vi "DriveStateController.vi"(1 "Selected State (In)":string) -> (0 "Selected State (Out)":string)   [LabVIEW 2019]
doc: "This VI performs all of the calculations and decisions related to the swerve drive."
uses:
  <vilib>/Rock Robotics/WPI/DriverStation/WPI_DriverStationRobotMode2.ctl
  dsinstructions.vi
  constants.vi
  dsdata.vi
  sensors.vi
  outputs.vi
panel:
  in  "Deceleration Hysteresis (ms)":u32
  in  "Driver Profiles":T1(array[cluster])=[{"Strafe Deadband"=0.08, "Rotation Deadband"=0.15, "Strafe Scaling"=3.0, "Rotation Scaling"=2.5}, {"Strafe Deadband"=0.08, "Rotation Deadband"=0.15, "Strafe Scaling"=2.0, "Rotation Scaling"=2.5}, {"Strafe Deadband"=0.08, "Rotation Deadband"=0.15, "Strafe Scaling"=2.0, "Rotation Scaling"=2.5}, {"Strafe Deadband"=0.08, "Rotation Deadband"=0.15, "Strafe Scaling"=2.0, "Rotation Scaling"=2.5}] {"Rotation Scaling" min=1.0 max=4.0 scale=1.0..4.0; "Strafe Scaling" min=1.0 max=4.0 scale=1.0..4.0; "Rotation Deadband" min=0.0 max=0.4 scale=0.0..0.4; "Strafe Deadband" min=0.0 max=0.4 scale=0.0..0.4}
  out "Heading Control":bool
  in  "Heading Lock Strafe Deadband (ft/s)":dbl=1.0
  in  "PID Tuning Heading Lock":T2={"Kp"=0.009, "Ki"=0.0, "Kd"=0.0001, "N-Diff"=5, "N-Int"=10, "Int Error Window"=30.0, "Max Ouput"=1.0, "Min Output"=-1.0} {"Int Error Window" min=0.0; "N-Int" min=2; "N-Diff" min=2; "Kd" min=0.0; "Ki" min=0.0; "Kp" min=0.0}
  in  "Manually Disable Heading Lock":bool
  in  "PID Tuning Feeder Station":T2={"Kp"=0.01, "Ki"=0.01, "Kd"=9e-05, "N-Diff"=10, "N-Int"=10, "Int Error Window"=30.0, "Max Ouput"=1.0, "Min Output"=-1.0} {"Int Error Window" min=0.0; "N-Int" min=2; "N-Diff" min=2; "Kd" min=0.0; "Ki" min=0.0; "Kp" min=0.0}
  out "Heading Controller Summary":T3(graph)
  in  "PID Tuning Auto Targeting":T2={"Kp"=0.01, "Ki"=0.01, "Kd"=9e-05, "N-Diff"=10, "N-Int"=10, "Int Error Window"=30.0, "Max Ouput"=1.0, "Min Output"=-1.0} {"Int Error Window" min=0.0; "N-Int" min=2; "N-Diff" min=2; "Kd" min=0.0; "Ki" min=0.0; "Kp" min=0.0}
  in  "Manual Fudge Factor (deg)":dbl=5.0
  in  "Plot Heading PID":bool
  in  "Sync Driver Profile":bool
  out "Selected Driver":string
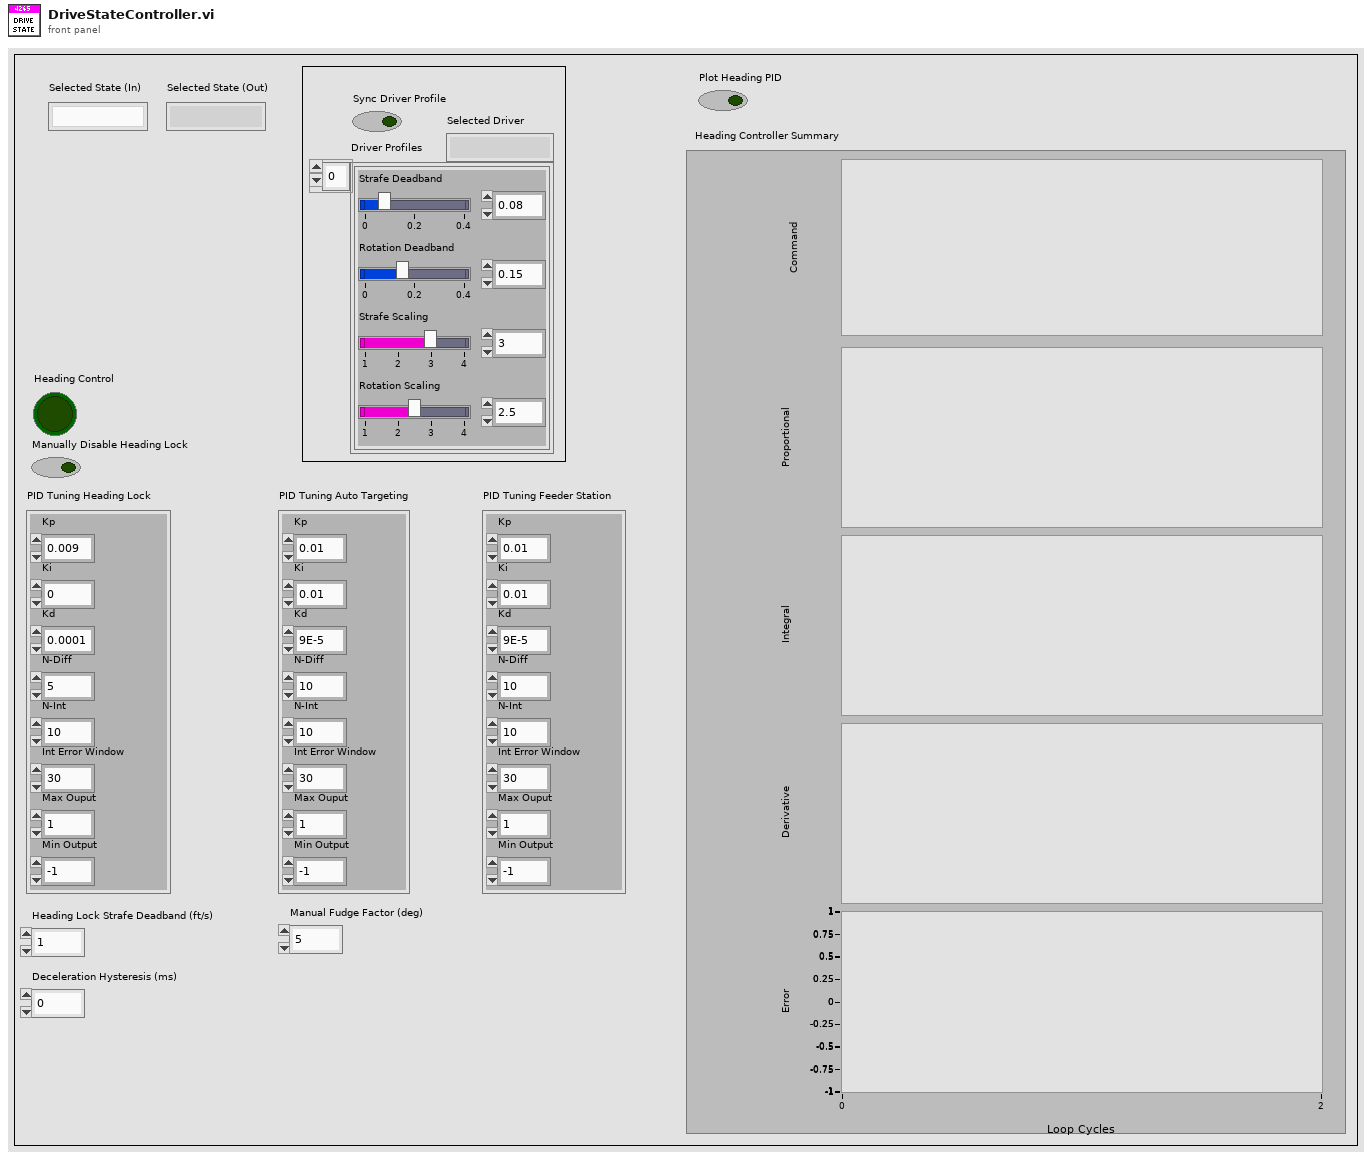
[diagram p1: front panel]
types:
  T1 = cluster{"Strafe Deadband":dbl, "Rotation Deadband":dbl, "Strafe Scaling":dbl, "Rotation Scaling":dbl}[]
  T2 = cluster{"Kp":dbl, "Ki":dbl, "Kd":dbl, "N-Diff":i32, "N-Int":i32, "Int Error Window":dbl, "Max Ouput":dbl, "Min Output":dbl}
  T3 = cluster{"Command":dbl, "Proportional":dbl, "Integral":dbl, "Derivative":dbl, "Goal":dbl}
  T4 = typedef "WPI_DriverStationRobotMode2.ctl" = enum16{"Autonomous Disabled", "Autonomous Enabled", "Teleop Disabled", "Teleop Enabled", "Disconnected", "Finish", "Test Disabled", "Test Enabled", "Emergency Stopped"}
  T5 = enum16{"Driver Control", "Auto Targeting", "Feeder Station"}
  T6 = cluster{"Strafe Deadband":dbl, "Rotation Deadband":dbl, "Strafe Scaling":dbl, "Rotation Scaling":dbl}
  T7 = enum16{"Center", "Module 0", "Module 1", "Module 2", "Module 3"}
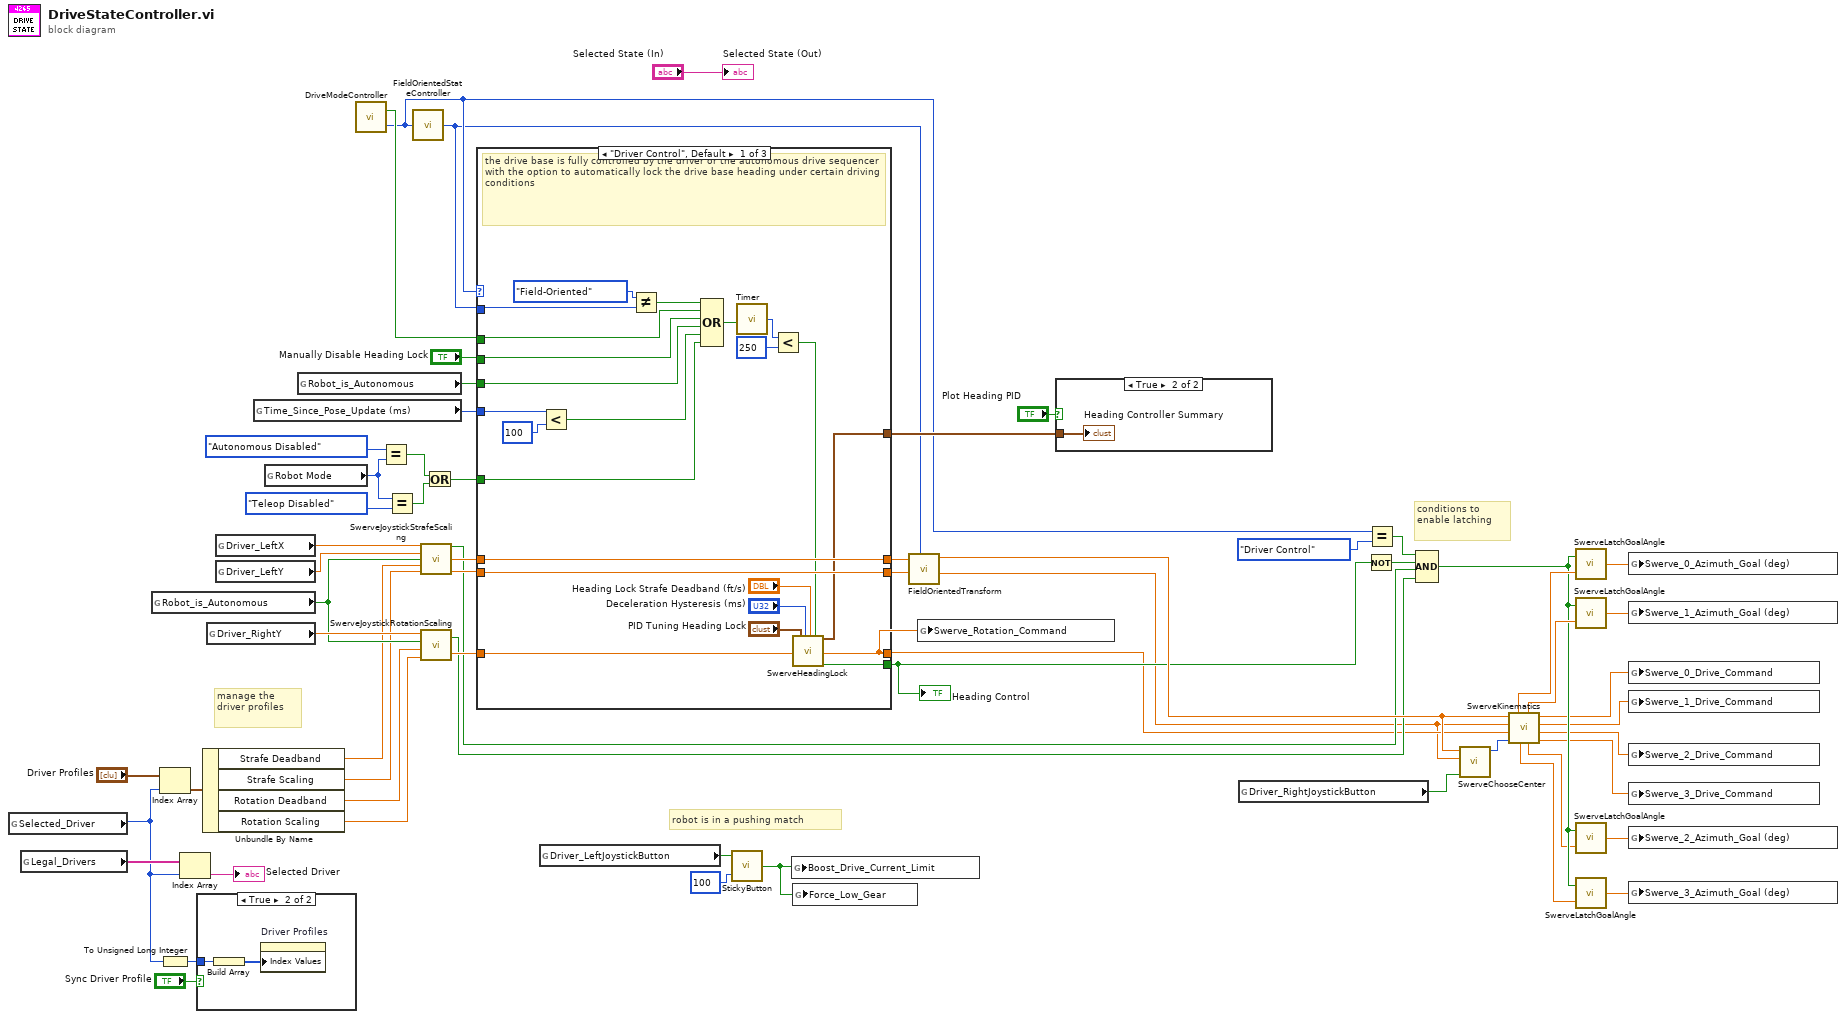
[diagram p0: block diagram]
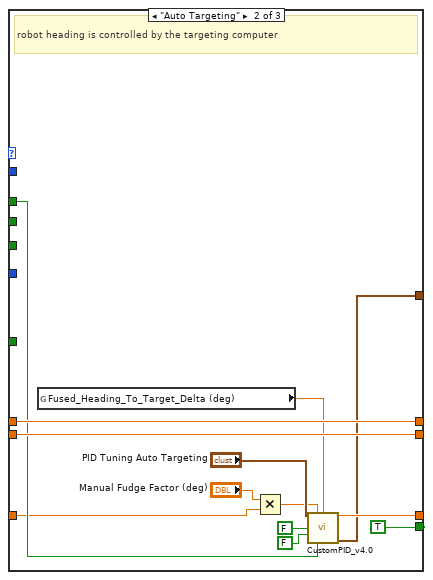
[diagram p3: hidden frame]
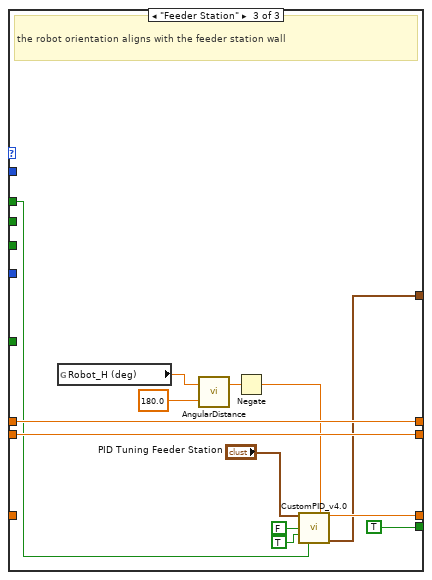
[diagram p4: hidden frame]
diagram:
  # "robot is in a pushing match"
  # "conditions to\nenable latching"
  # "manage the\ndriver profiles"
  n1 = global read "dsdata.vi" "Selected_Driver"() -> (w22:i32)
  n2 = global read "constants.vi" "Legal_Drivers"() -> (w56:string[])
  n3 = global read "dsdata.vi" "Robot_is_Autonomous"() -> (w36:bool)
  n4 = Index Array(array="Driver Profiles", index=w22) -> (element=w21:T6)
  n5 = To Unsigned Long Integer(number=w22) -> (unsigned 32bit integer=w58:u32)
  n6 = Index Array(array=w56, index=w22) -> (element=→"Selected Driver":string)
  n7 = case shown="True" "Sync Driver Profile" {
    tunnel: w58 -> [_ w64]
    frame False {
    }
    frame True {
      n8 = Build Array(w64) -> (w63:u32[])
      n9 = property on="Driver Profiles" class="Arr (strict)"("Index Values"=w63) -> ()  [unwired: 2 in, 2 out]
    }
  }
  n10 = Unbundle By Name(w21) -> ("Strafe Deadband"=w20:dbl, "Strafe Scaling"=w19:dbl, "Rotation Deadband"=w18:dbl, "Rotation Scaling"=w17:dbl)
  n11 = global read "dsinstructions.vi" "Driver_RightY"() -> (w37:dbl)
  n12 = global read "dsinstructions.vi" "Driver_LeftX"() -> (w42:dbl)
  n13 = global read "dsinstructions.vi" "Driver_LeftY"() -> (w41:dbl)
  n14 = global read "sensors.vi" "Time_Since_Pose_Update (ms)"() -> (w51:u32)
  n15 = global read "dsdata.vi" "Robot Mode"() -> (w6:T4)
  n16 = global read "dsdata.vi" "Robot_is_Autonomous"() -> (w50:bool)
  n17 = call "DriveModeController.vi"() -> ("Drive Mode Change"=w48:bool, "Drive Mode"=w28:T5)  [unwired: 1 in]
  n18 = Equal?(x=WPI_DriverStationRobotMode2."Autonomous Disabled" ("Robot Mode"), y=w6) -> (x = y?=w4:bool)
  n19 = Equal?(x=w6, y=WPI_DriverStationRobotMode2."Teleop Disabled" ("Robot Mode")) -> (x = y?=w3:bool)
  n20 = call "FieldOrientedStateController.vi"("Drive Mode"=w28) -> ("Orientation Mode"=w25:enum16{"Robot-Oriented", "Field-Oriented"})
  n21 = call "SwerveJoystickStrafeScaling.vi"("Raw Joystick X"=w42, "Raw Joystick Y"=w41, "Auto Control"=w36, "Strafe Deadband"=w20, "Strafe Scaling"=w19) -> ("In Deadband"=w32:bool, "Scaled Joystick X"=w40:dbl, "Scaled Joystick Y"=w39:dbl)  [unwired: 8 in]
  n22 = call "SwerveJoystickRotationScaling.vi"("Rotation Scaling"=w17, "Rotation Deadband"=w18, "Auto Control"=w36, "Raw Joystick Rotation"=w37) -> ("Scaled Joystick Rotation"=w38:dbl, "In Deadband"=w33:bool)
  n23 = Or(x=w4, y=w3) -> (x .or. y?=w2:bool)
  n24 = case shown="\"Driver Control\", Default" w28 {
    tunnel: [w83 w99 w111] -> w24
    tunnel: [w82 w100 w109] -> w62
    tunnel: w40 -> [w82 w100 w109]
    tunnel: w39 -> [w83 w99 w111]
    tunnel: w38 -> [w75 w89 _]
    tunnel: [w76 w91 w108] -> w31
    tunnel: [w81 TRUE ("auto rot control") TRUE ("auto rot control")] -> w34
    tunnel: w25 -> [w84 _ _]
    tunnel: w50 -> [w79 _ _]
    tunnel: w48 -> [w72 w94 w104]
    tunnel: w51 -> [w87 _ _]
    tunnel: [w78 w90 w103] -> w49
    tunnel: "Manually Disable Heading Lock" -> [w77 _ _]
    tunnel: w2 -> [w66 _ _]
    frame "Driver Control", Default {
      # "the drive base is fully controlled by the driver or the autonomous drive sequencer with the option to automatically lock the drive base heading under certain driving conditions"
      n25 = Less?(x=w87, y=u32 100) -> (x < y?=w80:bool)
      n26 = Not Equal?(x=enum16{"Robot-Oriented", "Field-Oriented"}."Field-Oriented" ("Orientation Mode"), y=w84) -> (x != y?=w71:bool)
      n27 = Compound Arithmetic op=OR(w71, w72, w77, w79, w80, w66) -> (w69:bool)
      n28 = call "Timer.vi"("Reset Timer"=w69) -> ("Time (ms)"=w70:u32)
      n29 = Less?(x=w70, y=u32 250) -> (x < y?=w67:bool)
      n30 = call "SwerveHeadingLock.vi"("Driver Rotation Joystick"=w75, "PID Tuning Parameters"="PID Tuning Heading Lock", "Deceleration Hysteresis (ms)"="Deceleration Hysteresis (ms)", "Heading Lock Strafe Deadband (ft/s)"="Heading Lock Strafe Deadband (ft/s)", "External Disables"=w67) -> ("Controller Summary"=w78:T3, "Joystick Rotation"=w76:dbl, "Heading Lock"=w81:bool)  [unwired: 12 in]
    }
    frame "Auto Targeting" {
      # "robot heading is controlled by the targeting computer"
      n31 = global read "sensors.vi" "Fused_Heading_To_Target_Delta (deg)"() -> (w95:dbl)
      n32 = Multiply(x="Manual Fudge Factor (deg)", y=w89) -> (x*y=w96:dbl)
      n33 = call "CustomPID_v4.0.vi"("PID Tuning Parameters"="PID Tuning Auto Targeting", "Goal"=w96, "Process Variable"=w95, "Reset on Goal Change ?"=FALSE, "Use Custom Error Calculation ?"=FALSE, "Reinit"=w94) -> ("Command"=w91:dbl, "Controller Summary"=w90:T3)  [unwired: 6 in, 2 out]
    }
    frame "Feeder Station" {
      # "the robot orientation aligns with the feeder station wall"
      n34 = global read "sensors.vi" "Robot_H (deg)"() -> (w113:dbl)
      n35 = call "AngularDistance.vi"("Goal Angle (deg) [0,360]"=180.0, "Current Angle (deg) [-Inf,+Inf]"=w113) -> ("Signed Angular Distance (deg) [-180,+180]"=w102:dbl)  [unwired: 1 out]
      n36 = Negate(x=w102) -> (-x=w101:dbl)
      n37 = call "CustomPID_v4.0.vi"("PID Tuning Parameters"="PID Tuning Feeder Station", "Custom Error Calculation"=w101, "Reset on Goal Change ?"=FALSE, "Use Custom Error Calculation ?"=TRUE, "Reinit"=w104) -> ("Command"=w108:dbl, "Controller Summary"=w103:T3)  [unwired: 7 in, 2 out]
    }
  }
  "Heading Control" <- w34
  n38 = global read "dsinstructions.vi" "Driver_LeftJoystickButton"() -> (w44:bool)
  n39 = call "StickyButton.vi"("Time threshold (ms)"=u32 100 ("y"), "Button Input"=w44) -> ("Sticky Button"=w1:bool)
  n40 = global write "outputs.vi" "Boost_Drive_Current_Limit"(w1) -> ()
  n41 = global write "outputs.vi" "Force_Low_Gear"(w1) -> ()
  n42 = call "FieldOrientedTransform.vi"("Orientation Mode"=w25, "Joystick Y"=w24, "Joystick X"=w62) -> ("Joystick Y'"=w26:dbl, "Joystick X'"=w35:dbl)  [unwired: 7 in]
  n43 = global write "outputs.vi" "Swerve_Rotation_Command"(w31) -> ()
  n44 = case shown="True" "Plot Heading PID" {
    tunnel: w49 -> [_ w114]
    frame False {
    }
    frame True {
      "Heading Controller Summary" <- w114
    }
  }
  n45 = global read "dsinstructions.vi" "Driver_RightJoystickButton"() -> (w47:bool)
  n46 = Not(x=w34) -> (.not. x?=w30:bool)
  n47 = Equal?(x=w28, y=T5."Driver Control" ("x")) -> (x = y?=w29:bool)
  n48 = Compound Arithmetic op=AND(w29, w30, w32, w33) -> (w54:bool)
  n49 = call "SwerveChooseCenter.vi"("Defensive Driving Trigger"=w47, "Joystick Y"=w26, "Joystick X"=w35) -> ("Center Choice"=w46:T7)  [unwired: 6 in]
  n50 = call "SwerveKinematics.vi"("Rotation Center Choice"=w46, "Joystick Rotation"=w31, "Joystick Y"=w26, "Joystick X"=w35) -> ("Module 3 Velocity Command (ul)"=w12:dbl, "Module 2 Velocity Command (ul)"=w13:dbl, "Module 1 Velocity Command (ul)"=w14:dbl, "Module 0 Velocity Command (ul)"=w15:dbl, "Module 2 Angle (deg)"=w53:dbl, "Module 1 Angle (deg)"=w60:dbl, "Module 3 Angle (deg)"=w52:dbl, "Module 0 Angle (deg)"=w61:dbl)
  n51 = call "SwerveLatchGoalAngle.vi"("Raw Goal Angle"=w61, "In Deadband"=w54) -> ("Latched Goal Angle"=w11:dbl)
  n52 = call "SwerveLatchGoalAngle.vi"("Raw Goal Angle"=w60, "In Deadband"=w54) -> ("Latched Goal Angle"=w10:dbl)
  n53 = call "SwerveLatchGoalAngle.vi"("Raw Goal Angle"=w53, "In Deadband"=w54) -> ("Latched Goal Angle"=w9:dbl)
  n54 = call "SwerveLatchGoalAngle.vi"("Raw Goal Angle"=w52, "In Deadband"=w54) -> ("Latched Goal Angle"=w8:dbl)
  n55 = global write "outputs.vi" "Swerve_0_Azimuth_Goal (deg)"(w11) -> ()
  n56 = global write "outputs.vi" "Swerve_1_Azimuth_Goal (deg)"(w10) -> ()
  n57 = global write "outputs.vi" "Swerve_0_Drive_Command"(w15) -> ()
  n58 = global write "outputs.vi" "Swerve_1_Drive_Command"(w14) -> ()
  n59 = global write "outputs.vi" "Swerve_2_Drive_Command"(w13) -> ()
  n60 = global write "outputs.vi" "Swerve_3_Drive_Command"(w12) -> ()
  n61 = global write "outputs.vi" "Swerve_2_Azimuth_Goal (deg)"(w9) -> ()
  n62 = global write "outputs.vi" "Swerve_3_Azimuth_Goal (deg)"(w8) -> ()
  "Selected State (Out)" <- "Selected State (In)"
